vi "Validate Routing Channels or Folder Reference.vi"(8 "error in":errorcluster, 11 "routing channels in":T1 format="%.0x") -> (0 "error out":errorcluster, 3 "routing channels out":T1 format="%.0x")   [LabVIEW 2017, in "Routing and Faulting Scripting.lvlib"]
uses:
  Routing and Faulting Scripting.lvlib
  <vilib>/NI Veristand/Custom Device API/Custom Device Item Ref.ctl
  Shared/Constants.vi
  Shared/Routing and Faulting Shared.lvlib
  <vilib>/NI Veristand/Custom Device API/Custom Device API.lvlib
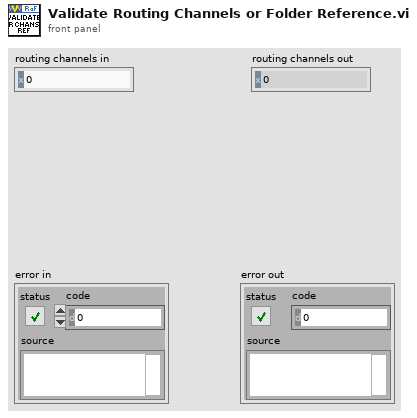
[diagram p1: front panel]
types:
  T1 = typedef "Custom Device API.lvlib/Custom Device Item Ref.ctl" = u64
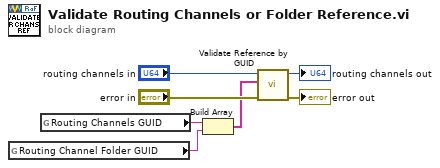
[diagram p0: block diagram]
diagram:
  n1 = global read "Constants.vi" "Routing Channel Folder GUID"() -> (w2:string)
  n2 = global read "Constants.vi" "Routing Channels GUID"() -> (w3:string)
  n3 = Build Array(w3, w2) -> (w1:string[])
  n4 = call "Validate Reference by GUID.vi"("error in"="error in", "valid guids"=w1, "item in"="routing channels in") -> ("error out"=→"error out":errorcluster, "item out"=→"routing channels out":T1)  [unwired: 7 in]
